vi "Heartbeat.vi"(8 "error in (no error)":errorcluster, 11 "PLC_Module in":refnum<class "PLC_Module.lvclass">) -> (0 "error out":errorcluster, 3 "PLC_Module out":refnum<class "PLC_Module.lvclass">)   [LabVIEW 2025, in "PLC_Module.lvlib" / "PLC_Module.lvclass"]
uses:
  PLC_Module.lvclass
  PLC_Module.lvclass/PLC_Module.ctl
  32c81189-79d1-488a-b42c-1dacc65e9abb.vi
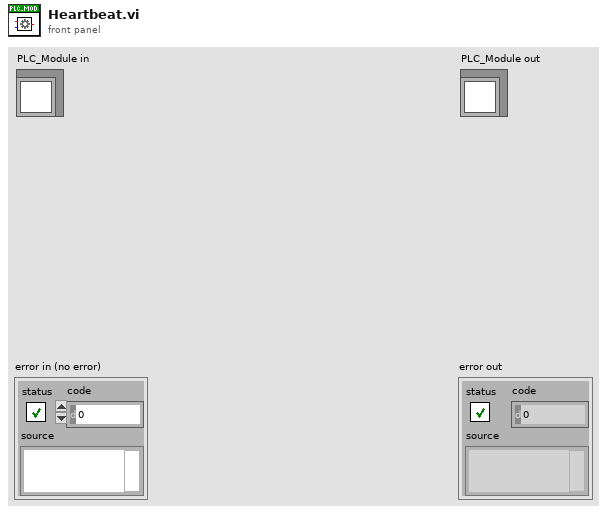
[diagram p1: front panel]
types:
  T1 = typedef "PLC_Module.lvlib/PLC_Module.lvclass/PLC_Data_Config.ctl" = map{string, cluster{"Config":T2, "Get Value":string, "Set Value":string}}
  T2 = typedef "PLC_Module.lvlib/PLC_Module.lvclass/PLC_Data.ctl" = cluster{"Address":string, "Direction":enum16{"PC->PLC", "PLC->PC"}, "DataType":T3, "Description":string}
  T3 = typedef "PLC_Module.lvlib/PLC_Module.lvclass/PLC_Data_Type.ctl" = enum16{"Boolean", "Single Float", "U8", "U32", "U32_Array", "String"}
  T4 = cluster{"Config":T2, "Get Value":string, "Set Value":string}
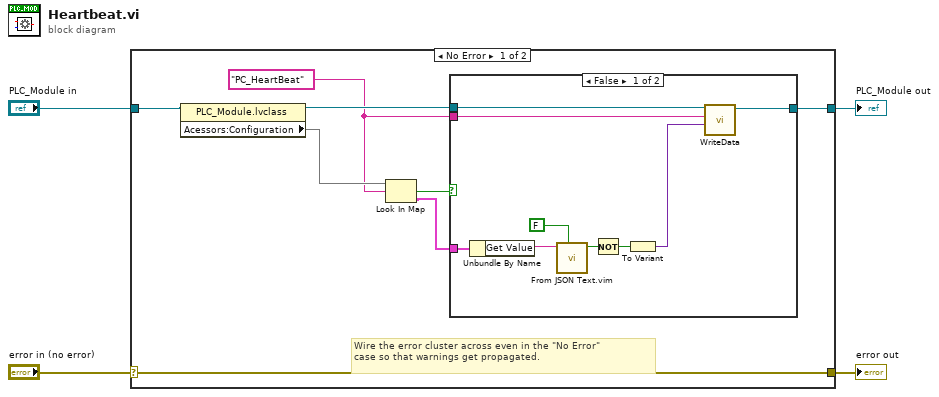
[diagram p0: block diagram]
diagram:
  n1 = case shown="No Error" "error in (no error)" {
    selector: "error in (no error)" -> [w12 w24]
    tunnel: [w12 w24] -> w3
    tunnel: [w11 w23] -> w1
    tunnel: "PLC_Module in" -> [w10 w23]
    frame No Error {
      w7 = "PC_HeartBeat" ("key")
      # "Wire the error cluster across even in the \"No Error\"\ncase so that warnings get propagated."
      n2 = property class="PLC_Module.lvclass"(reference=w10) -> (reference out=w9:refnum<class "PLC_Module.lvclass">, "Acessors:Configuration"=w8:T1)  [unwired: 1 in, 1 out]
      n3 = Look In Map(map=w8, key=w7) -> (key not found?=w5:bool, value=w6:T4)  [unwired: 1 in]
      n4 = case shown="False" w5 {
        tunnel: [w21 w22] -> w11
        tunnel: w9 -> [w20 w22]
        tunnel: w7 -> [w17 _]
        tunnel: w6 -> [w16 _]
        frame False {
          n5 = Unbundle By Name(w16) -> ("Get Value"=w19:string)
          n6 = call "From JSON Text.vim"("Data Type and Default Value"=FALSE, "JSON"=w19) -> ("Data out"=w15:bool)  [unwired: 8 in, 1 out]
          n7 = Not(x=w15) -> (.not. x?=w14:bool)
          n8 = To Variant(anything=w14) -> (Variant=w13:variant)
          n9 = call "WriteData.vi"("Data"=w13, "LogicName"=w17, "PLC_Module in"=w20) -> ("PLC_Module out"=w21:refnum<class "PLC_Module.lvclass">)  [unwired: 7 in, 1 out]
        }
        frame True {
        }
      }
    }
    frame Error {
    }
  }
  "error out" <- w3
  "PLC_Module out" <- w1
